vi "S7_1200 Read.vi"   [LabVIEW 2020, in "S7_1200 control.lvlib"]
uses:
  S7_1200 control.lvlib
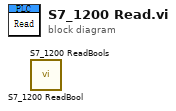
[diagram p0: block diagram]
diagram:
  n1 = call "S7_1200 ReadBool.vi"() -> ()  [unwired: 5 in, 3 out]
  n2 = call "S7_1200 ReadBools.vi"() -> ()  [unwired: 5 in, 3 out]
